vi "Liam - Manual Assembly Test.vi"() -> ()   [LabVIEW 2020]
uses:
  Classes/Assembly/Assembly Run.lvclass
  Classes/Workspace/Fixture Enum.ctl
  Classes/Workspace/Fixture.lvclass
  Classes/Controller/Controller.lvclass
  Classes/Routine/Routine Enum.ctl
  Classes/Routine/Routine.lvclass
panel:
  in  "Remove":bool
  in  "Stage":i32(listbox)=-1
  in  "Add":bool
  in  "Routine":T1=enum."Dispense on Plate"
  in  "Update":bool
  in  "Stop":bool
  in  "Go":bool
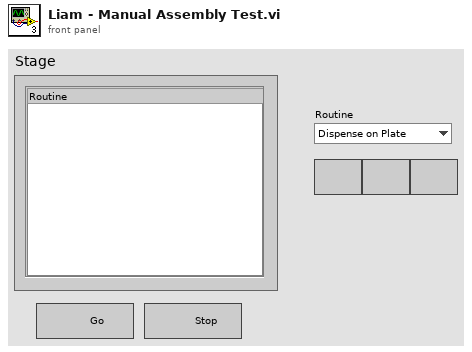
[diagram p1: front panel]
types:
  T1 = typedef "Routine.lvclass/Routine Enum.ctl" = enum16{"Primary Pick Up", "Pick Up All", "Put Down Secondary", "Put Down All", "Release Syringe", "Secondary Pick Up", "Secure Syringe", "Dispense on Plate", "Dispense on Kapton", "Dispense on Sensor"}
  T2 = typedef "Fixture.lvclass/Fixture Enum.ctl" = enum16{"Assembly Tray", "Syringe Space", "Component", "Pick Up Tool", "Current Position"}
  T3 = typedef "Controller.lvclass/Controllers.ctl" = cluster{"I-O.lvclass":refnum<class "I-O.lvclass">, "Gantry":refnum<k24>, "Dispenser":refnum<visa-resource-name>}
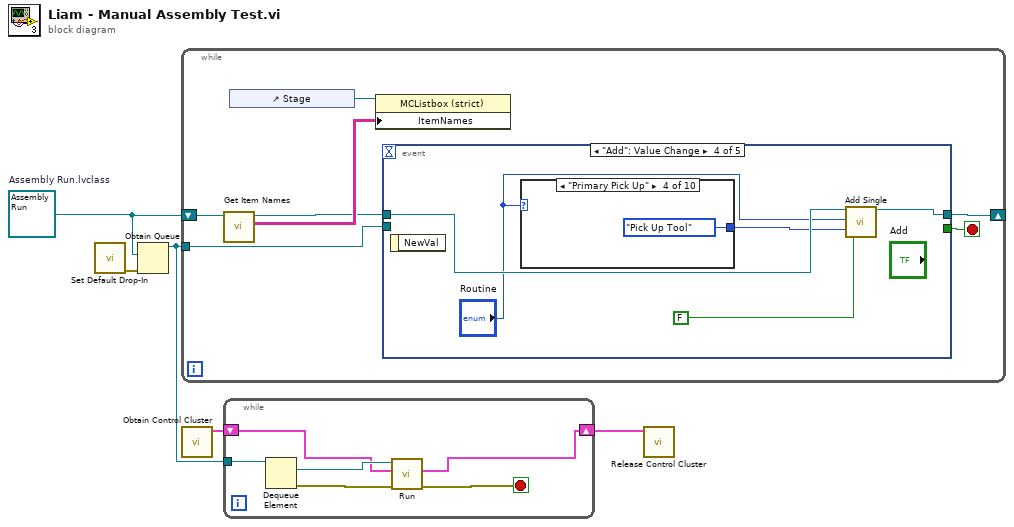
[diagram p0: block diagram]
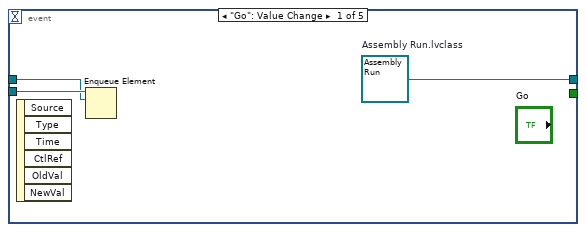
[diagram p2: hidden frame]
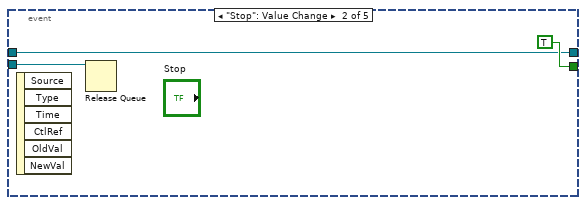
[diagram p3: hidden frame]
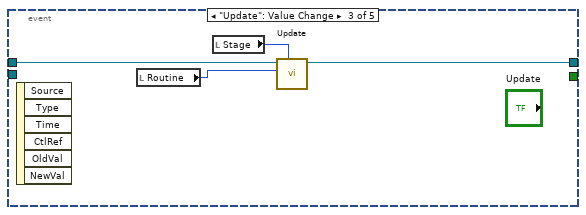
[diagram p4: hidden frame]
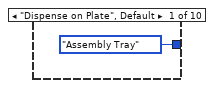
[diagram p5: hidden frame]
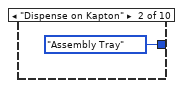
[diagram p6: hidden frame]
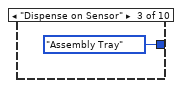
[diagram p7: hidden frame]
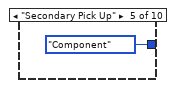
[diagram p8: hidden frame]
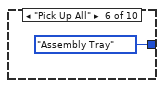
[diagram p9: hidden frame]
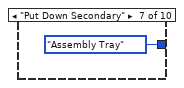
[diagram p10: hidden frame]
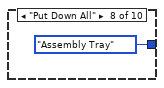
[diagram p11: hidden frame]
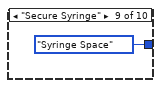
[diagram p12: hidden frame]
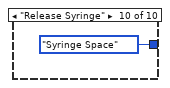
[diagram p13: hidden frame]
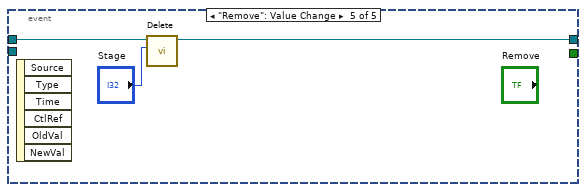
[diagram p14: hidden frame]
diagram:
  w1 = refnum<class "Assembly Run.lvclass"> refnum  # Assembly Run.lvclass
  n1 = call "Set Default Drop-In.vi"() -> ("error out"=w2:errorcluster)  [unwired: 11 in]
  n2 = Obtain Queue(element data type=w1, error in (no error)=w2) -> (queue out=w5:refnum<queue>)  [unwired: 3 in, 2 out]
  n3 = while {
    shift-right: [w6] -> _
    shift-left: w1 -> [w8]
    tunnel: w5 -> [w11]
    stop <- w12 stop-if-true
    n4 = call "Get Item Names.vi"("Assembly Run in"=w8) -> ("Item names"=w10:string[][], "Assembly Run out"=w7:refnum<class "Assembly Run.lvclass">)  [unwired: 8 in, 1 out]
    n5 = control-ref of="Stage"() -> (w9:refnum<vi>)
    n6 = property class="MCListbox (strict)"(reference=w9, "ItemNames"=w10) -> ()  [unwired: 1 in, 2 out]
    n7 = event shown="[3] \"Add\": Value Change" {
      selector: _ -> [_ _ _ _ _]
      dyn-events: _ -> [_ _ _ _ _]
      timeout: _ -> [_ _ _ _ _]
      tunnel: [_ TRUE _ _ _] -> w12
      tunnel: w7 -> [w14 w17 w22 w27 w40]
      tunnel: [w13 w17 w21 w26 w39] -> w6
      tunnel: w11 -> [w15 w16 _ _ _]
      event "Go": Value Change {
        w13 = refnum<class "Assembly Run.lvclass"> refnum  # Assembly Run.lvclass
        n8 = event-data() -> ()  [unwired: 1 in, 6 out]
        n9 = Enqueue Element(queue=w15, element=w14) -> ()  [unwired: 2 in, 3 out]
      }
      event "Stop": Value Change {
        n10 = event-data() -> ()  [unwired: 1 in, 6 out]
        n11 = Release Queue(queue=w16) -> ()  [unwired: 2 in, 3 out]
      }
      event "Update": Value Change {
        n12 = event-data() -> ()  [unwired: 1 in, 6 out]
        n13 = local read "Routine"() -> (w20:T1)
        n14 = local read "Stage"() -> (w19:i32)
        n15 = call "Update.vi"("Row"=w19, "Routine"=w20, "Assembly Run in"=w22) -> ("Assembly Run out"=w21:refnum<class "Assembly Run.lvclass">)  [unwired: 7 in, 1 out]
      }
      event "Add": Value Change {
        n16 = event-data() -> ()  [unwired: 1 in, 1 out]
        n17 = case shown="\"Primary Pick Up\"" "Routine" {
          tunnel: [Fixture_Enum."Assembly Tray" ("Fixture") Fixture_Enum."Assembly Tray" ("Fixture") Fixture_Enum."Assembly Tray" ("Fixture") Fixture_Enum."Pick Up Tool" ("Fixture") Fixture_Enum."Component" ("Fixture") Fixture_Enum."Assembly Tray" ("Fixture") Fixture_Enum."Assembly Tray" ("Fixture") Fixture_Enum."Assembly Tray" ("Fixture") Fixture_Enum."Syringe Space" ("Fixture") Fixture_Enum."Syringe Space" ("Fixture")] -> w25
          frame "Dispense on Plate", Default {
          }
          frame "Dispense on Kapton" {
          }
          frame "Dispense on Sensor" {
          }
          frame "Primary Pick Up" {
          }
          frame "Secondary Pick Up" {
          }
          frame "Pick Up All" {
          }
          frame "Put Down Secondary" {
          }
          frame "Put Down All" {
          }
          frame "Secure Syringe" {
          }
          frame "Release Syringe" {
          }
        }
        n18 = call-dynamic "Add Single.vi"("UI in"=w27, "Routine"="Routine", "Fixture"=w25, "Module Size"=FALSE) -> ("UI out"=w26:refnum<class "Assembly Run.lvclass">)  [unwired: 14 in, 1 out]
      }
      event "Remove": Value Change {
        n19 = event-data() -> ()  [unwired: 1 in, 6 out]
        n20 = call "Delete.vi"("Index"="Stage", "Assembly In"=w40) -> ("Assembly Out"=w39:refnum<class "Assembly Run.lvclass">)  [unwired: 8 in, 1 out]
      }
    }
  }
  n21 = call "Obtain Control Cluster.vi"() -> ("Control Out"=w4:T3)  [unwired: 11 in]
  n22 = while {
    tunnel: w5 -> [w46]
    shift-right: [w41] -> w3
    shift-left: w4 -> [w44]
    stop <- w42 stop-if-true
    n23 = Dequeue Element(queue=w46) -> (element=w45:refnum<class "Assembly Run.lvclass">, error out=w43:errorcluster)  [unwired: 2 in, 2 out]
    n24 = call-dynamic "Run.vi"("error in (no error)"=w43, "Control In"=w44, "Assembly In"=w45) -> ("error out"=w42:errorcluster, "Control Out"=w41:T3)  [unwired: 6 in, 1 out]
  }
  n25 = call "Release Control Cluster.vi"("output cluster"=w3) -> ()  [unwired: 11 in]
